vi "CursorDrag.vi"() -> ()   [LabVIEW 2012]
uses:
  <vilib>/Utility/miscctls.llb/LVPointDoubleTypeDef.ctl
  <vilib>/Utility/miscctls.llb/LVCursorListTypeDef.ctl
  <vilib>/measure/NI_MABase.lvlib
panel:
  out "游标位置":T1
  in  "sampling info":cluster{"Fs":dbl, "#s":dbl}={"Fs"=1000.0, "#s"=1000.0} caption="采样信息" {"Fs" format="%.2p"}
  out "游标列表":T2
  in  "停止":bool
  out "游标.游标位置":T1
  out "波形图":dbl[](graph)
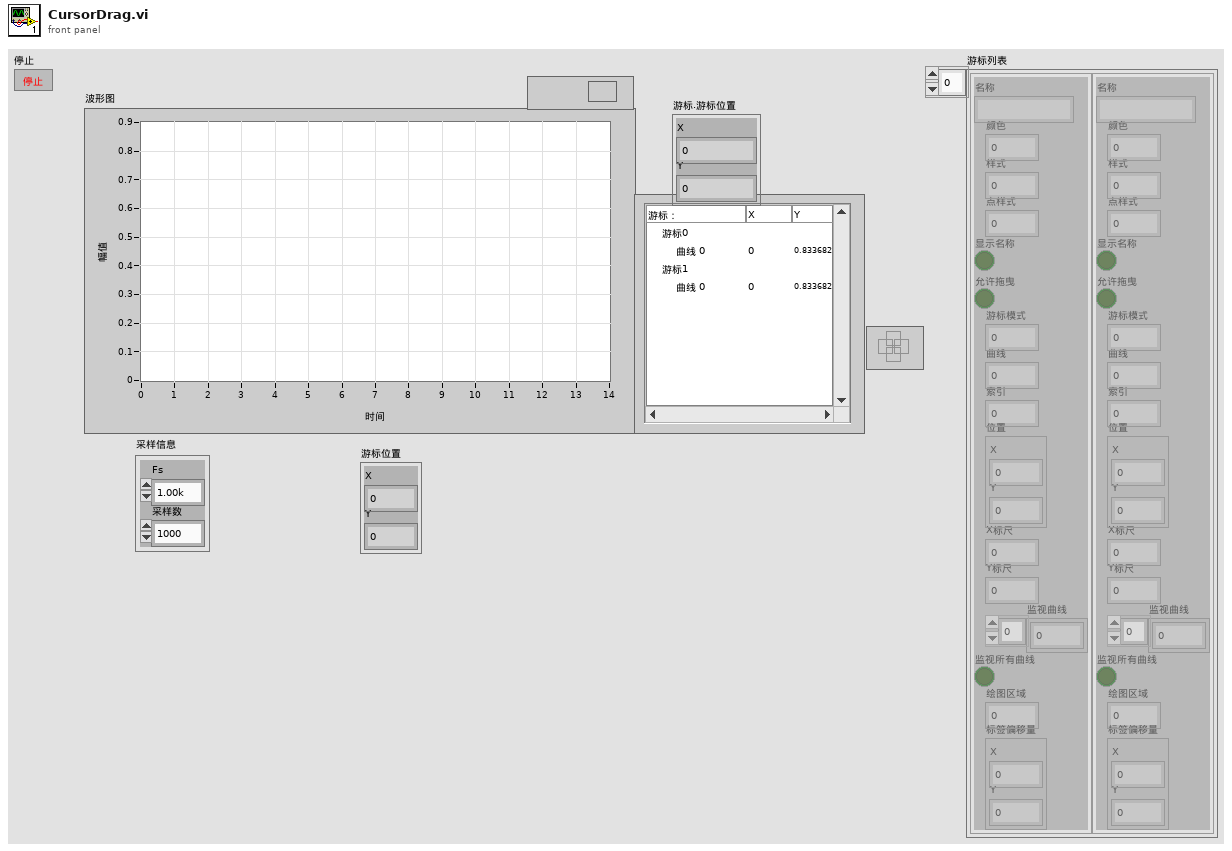
[diagram p1: front panel]
types:
  T1 = typedef "LVPointDoubleTypeDef.ctl" = cluster{"X":dbl, "Y":dbl}
  T2 = typedef "LVCursorListTypeDef.ctl" = cluster{"Name":string, "Color":u32, "Style":u8, "Point Style":u8, "Name Visible":bool, "Allow Drag":bool, "Cursor Mode":u32, "Plot":i32, "Index":i32, "Position":cluster{"X":dbl, "Y":dbl}, "X Scale":u32, "Y Scale":u32, "Watch Plots":i32[], "Watch All Plots":bool, "Plot Area":i32, "Label Offset":cluster{"X":dbl, "Y":dbl}}[]
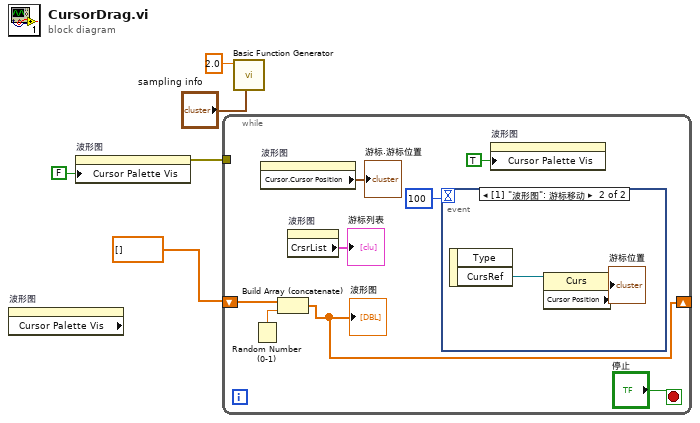
[diagram p0: block diagram]
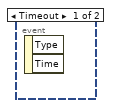
[diagram p2: hidden frame]
diagram:
  n1 = property on="波形图" class="WFGraph (严格)" props=["Cursor Palette Vis"]() -> ()  [unwired: 2 in, 3 out]
  n2 = property on="波形图" class="WFGraph (严格)"("Cursor Palette Vis"=FALSE ("游标图例可见")) -> (error out=w1:errorcluster)  [unwired: 2 in, 1 out]
  n3 = while {
    shift-right: [w7] -> _
    shift-left: dbl[] [] -> [w9]
    tunnel: w1 -> [_]
    stop <- "停止" stop-if-true
    n4 = Random Number (0-1)() -> (number: 0 to 1=w8:dbl)
    n5 = property on="波形图" class="WFGraph (严格)"() -> ("Cursor.Cursor Position"=→"游标.游标位置":T1)  [unwired: 2 in, 2 out]
    n6 = Build Array (concatenate)(w9, w8) -> (w7:dbl[])
    "波形图" <- w7
    n7 = property on="波形图" class="WFGraph (严格)"() -> ("CrsrList"=→"游标列表":T2)  [unwired: 2 in, 2 out]
    n8 = event shown="[1] \"波形图\": 游标移动" {
      selector: _ -> [_ _]
      dyn-events: _ -> [_ _]
      timeout: 100 -> [_ _]
      event Timeout {
        n9 = event-data() -> ()  [unwired: 1 in, 2 out]
      }
      event "波形图": Cursor Move {
        n10 = event-data() -> ("CursRef"=w15:refnum<vi>)  [unwired: 1 in, 1 out]
        n11 = property class="Curs"(reference=w15) -> ("Cursor Position"=→"游标位置":T1)  [unwired: 1 in, 2 out]
      }
    }
    n12 = property on="波形图" class="WFGraph (严格)"("Cursor Palette Vis"=TRUE ("游标图例可见")) -> ()  [unwired: 2 in, 2 out]
  }
  n13 = call <vilib>:"Basic Function Generator.vi"("sampling info"="sampling info", "frequency"=2.0) -> ()  [unwired: 7 in, 3 out]
